vi "UnitVector.vi"(9 "Vector 2":dbl[](array[numeric]), 10 "Vector 1":dbl[](array[numeric])) -> (2 "Unit Vector":dbl[](array[numeric]))   [LabVIEW 2010]
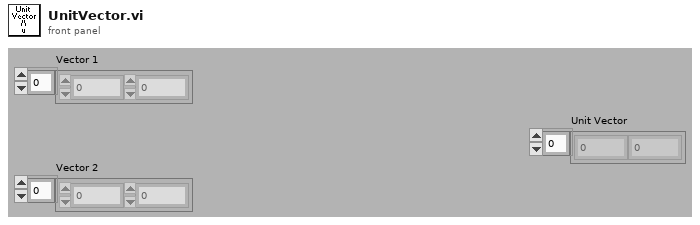
[diagram p1: front panel]
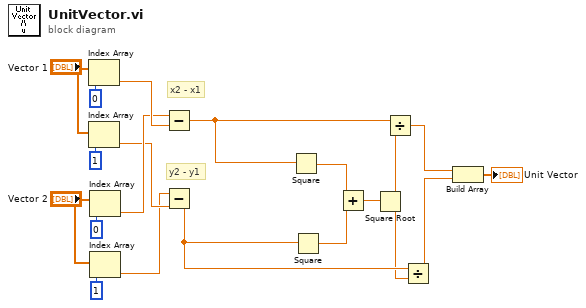
[diagram p0: block diagram]
diagram:
  # "y2 - y1"
  # "x2 - x1"
  n1 = Index Array(array="Vector 1", index=0) -> (element=w13:dbl)
  n2 = Index Array(array="Vector 1", index=1) -> (element=w11:dbl)
  n3 = Index Array(array="Vector 2", index=0) -> (element=w12:dbl)
  n4 = Index Array(array="Vector 2", index=1) -> (element=w10:dbl)
  n5 = Subtract(x=w12, y=w13) -> (x-y=w6:dbl)
  n6 = Subtract(x=w10, y=w11) -> (x-y=w5:dbl)
  n7 = Square(x=w6) -> (x^2=w9:dbl)
  n8 = Square(x=w5) -> (x^2=w8:dbl)
  n9 = Add(x=w9, y=w8) -> (x+y=w7:dbl)
  n10 = Square Root(x=w7) -> (sqrt(x)=w4:dbl)
  n11 = Divide(x=w6, y=w4) -> (x/y=w3:dbl)
  n12 = Divide(x=w5, y=w4) -> (x/y=w2:dbl)
  n13 = Build Array(w3, w2) -> (→"Unit Vector":dbl[])
